vi "Robot Systems.vi"(11 "Robot Commands":T1) -> ()   [LabVIEW 2014]
uses:
  Joystick/Robot Commands.ctl
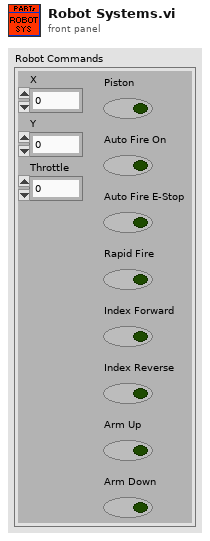
[diagram p1: front panel]
types:
  T1 = typedef "Robot Commands.ctl" = cluster{"X":dbl, "Y ":dbl, "Throttle":dbl, "Piston":bool, "Auto Fire On":bool, "Auto Fire E-Stop":bool, "Rapid Fire":bool, "Index Forward":bool, "Index Reverse ":bool, "Arm Up":bool, "Arm Down":bool}
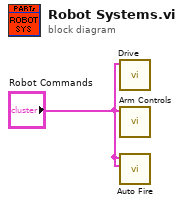
[diagram p0: block diagram]
diagram:
  n1 = call "Drive.vi"("Robot Commands"="Robot Commands") -> ()  [unwired: 10 in, 1 out]
  n2 = call "Arm Controls.vi"("Robot Commands"="Robot Commands") -> ()  [unwired: 11 in]
  n3 = call "Auto Fire.vi"("Robot Commands 2"="Robot Commands", "Robot Commands"="Robot Commands") -> ()  [unwired: 10 in]
